vi "serial_10.vi"(0 "VISA resource name":refnum<visa-resource-name>="COM4") -> ()   [LabVIEW 2010]
doc: "The Basic Serial Read and Write example performs a Serial Port Read, a Serial Port Write, or a combination of these actions. The user selects the actions (read or write) on the front panel. If both are selected, the VI will write the data first, read data, and then close the VISA session that is opened to the port. This VI will wait until the specified number of bytes is received at the port. Only the number of bytes specified will be read.\n\nINSTRUCTIONS:\n1) Select the serial resource and configuration parameters (baud rate, data bits, parity, stop bits, flow control).\n2) Select the operations to be performed. \n3) Connect the serial port to your device. If no device is available, perform a loopback test by doing one of the following. Short pins 2 and 3 on a RS-232 cable or short pin 4 to pin 8 and pin 5 to pin 9 on a RS-485/422 cable. \n4) Run the VI to see the data read. (The \"read string\" will match the \"string to write\" if a loopback test was performed.)\n\nNote: The parameters set for the serial port must match the parameters of the connected instrument or device. In this example, the bytes to read parameter specifies the number of bytes that the serial port reads. If there were more bytes at the port than the number specified in bytes to read, those bytes would not be read. Also, if you specify to read more bytes than the number of bytes actually read, you might receive a timeout error message.\n\nOn the block diagram, the Configure Serial Port VI sets the configuration parameters. The front panel displays the controls used to configure the basic parameters, such as baud rate, data bits, and parity. Constants configure the other parameters the user probably does not need set. After the VISA Configure Serial Port VI opens the VISA session and configures the port, the VI passes the VISA resource name to other VIs that perform operations on that VISA resource. The VISA Write function sends a command to the serial device and the VISA Read function returns data based on the command. The VISA Close function then closes the reference to the serial device. It is important to close the reference; otherwise communication through with that port through protocols other than VISA might not be possible."
panel:
  out "Sir citire intrari digitale":string
  out "Sem":dbl
  out "Leduri_com":bool[](array[boolean])
  out "Comutatoare":bool[](array[boolean])
  out "Comanda scriere iesiri digitale":string="O10"
  in  "Leduri":bool[](array[boolean])=[FALSE, FALSE, FALSE, FALSE, TRUE, FALSE, TRUE, FALSE]
  in  "Start":bool=TRUE
  # "Stop"
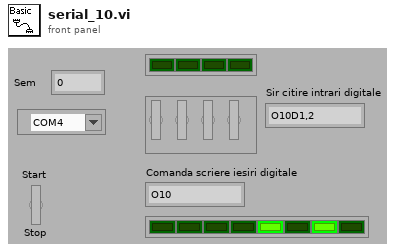
[diagram p1: front panel]
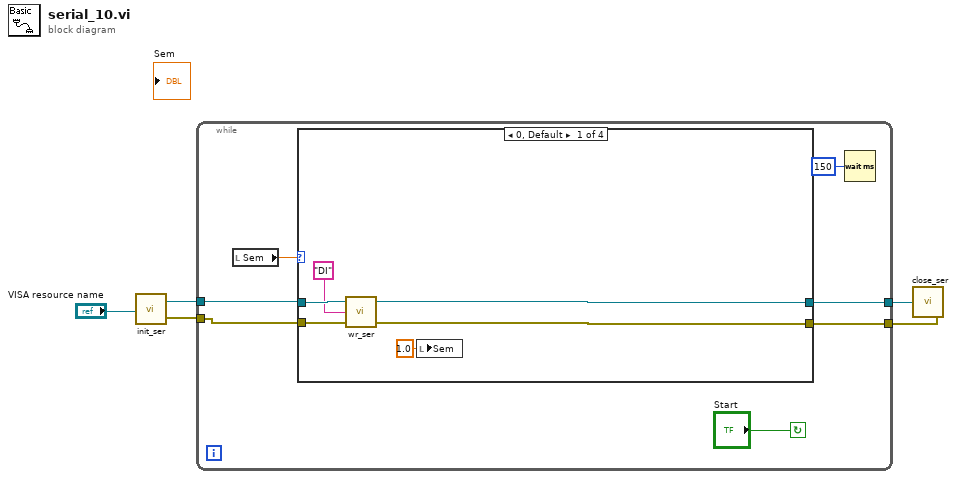
[diagram p0: block diagram]
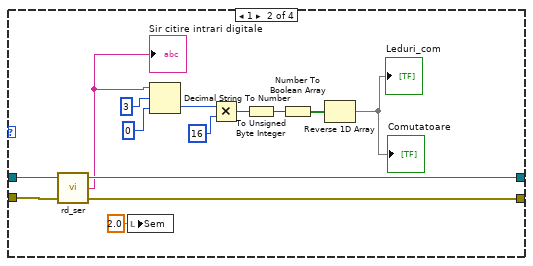
[diagram p2: hidden frame]
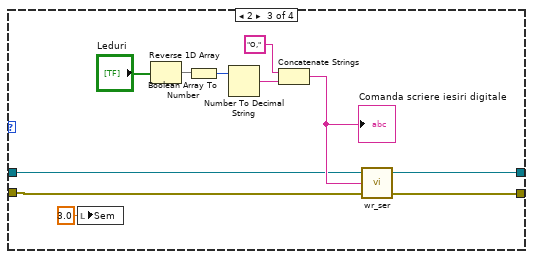
[diagram p3: hidden frame]
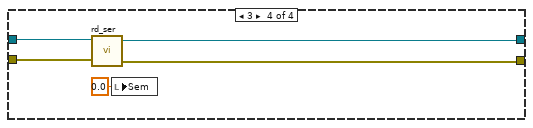
[diagram p4: hidden frame]
diagram:
  n1 = call "init_ser.vi"("VISA resource name"="VISA resource name") -> ("VISA resource name out"=w3:refnum<visa-resource-name>, "error out"=w4:errorcluster)
  n2 = while {
    tunnel: w4 -> [w7]
    tunnel: w3 -> [w8]
    tunnel: [w10] -> w2
    tunnel: [w9] -> w1
    stop <- "Start" continue-if-true
    n3 = local read "Sem"() -> (w11:dbl)
    n4 = case shown="0, Default" w11 {
      tunnel: w8 -> [w18 w32 w38 w48]
      tunnel: w7 -> [w17 w31 w37 w47]
      tunnel: [w15 w29 w35 w45] -> w9
      tunnel: [w16 w30 w36 w46] -> w10
      frame 0, Default {
        n5 = call "wr_ser.vi"("error in"=w17, "string to write"="DI", "VISA resource name in"=w18) -> ("error out"=w15:errorcluster, "VISA resource name out"=w16:refnum<visa-resource-name>)  [unwired: 1 in]
        n6 = local write "Sem"(1.0 ("Sem")) -> ()
      }
      frame 1 {
        n7 = call "rd_ser.vi"("error in"=w31, "VISA resource name in"=w32) -> ("error out"=w29:errorcluster, "read buffer"=w19:string, "VISA resource name out"=w30:refnum<visa-resource-name>)  [unwired: 1 in]
        "Sir citire intrari digitale" <- w19
        n8 = local write "Sem"(2.0 ("Sem")) -> ()
        n9 = Decimal String To Number(string=w19, offset=3, default (0L)=0) -> (number=w25:i32)  [unwired: 1 out]
        n10 = Multiply(x=w25, y=16) -> (x*y=w22:i32)
        n11 = To Unsigned Byte Integer(number=w22) -> (unsigned 8bit integer=w21:u8)
        n12 = Number To Boolean Array(number=w21) -> (Boolean array=w23:bool[])
        n13 = Reverse 1D Array(array=w23) -> (reversed array=→"Leduri_com" →"Comutatoare":bool[])
      }
      frame 2 {
        n14 = local write "Sem"(3.0 ("Sem")) -> ()
        n15 = Reverse 1D Array(array="Leduri") -> (reversed array=w42:bool[])
        n16 = Boolean Array To Number(Boolean array=w42) -> (number=w43:u32)
        n17 = Number To Decimal String(number=w43) -> (decimal integer string=w40:string)  [unwired: 1 in]
        n18 = Concatenate Strings("O,", w40) -> (w39:string)
        "Comanda scriere iesiri digitale" <- w39
        n19 = call "wr_ser.vi"("error in"=w37, "string to write"=w39, "VISA resource name in"=w38) -> ("error out"=w35:errorcluster, "VISA resource name out"=w36:refnum<visa-resource-name>)  [unwired: 1 in]
      }
      frame 3 {
        n20 = call "rd_ser.vi"("error in"=w47, "VISA resource name in"=w48) -> ("error out"=w45:errorcluster, "VISA resource name out"=w46:refnum<visa-resource-name>)  [unwired: 1 in, 1 out]
        n21 = local write "Sem"(0.0 ("Sem")) -> ()
      }
    }
    n22 = Wait (ms)(milliseconds to wait=u32 150) -> ()  [unwired: 1 out]
  }
  n23 = call "close_ser.vi"("error in"=w1, "VISA resource name in"=w2) -> ()
